vi "MetadataFromRD.vi"(9 "ChannelNames":string[](array[string]), 10 "ChannelName":string, 11 "Raw data file":path) -> (0 "allFound":bool, 1 "ValueStrings":string[](array[string]), 2 "ValueString":string, 4 "Name-Value Array":string[][](array[string]))   [LabVIEW 2021]
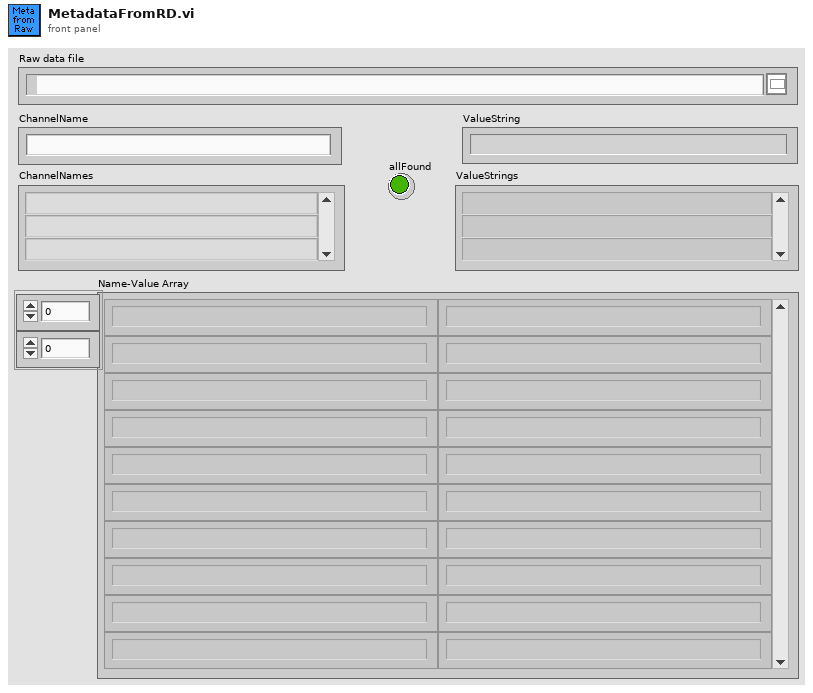
[diagram p1: front panel]
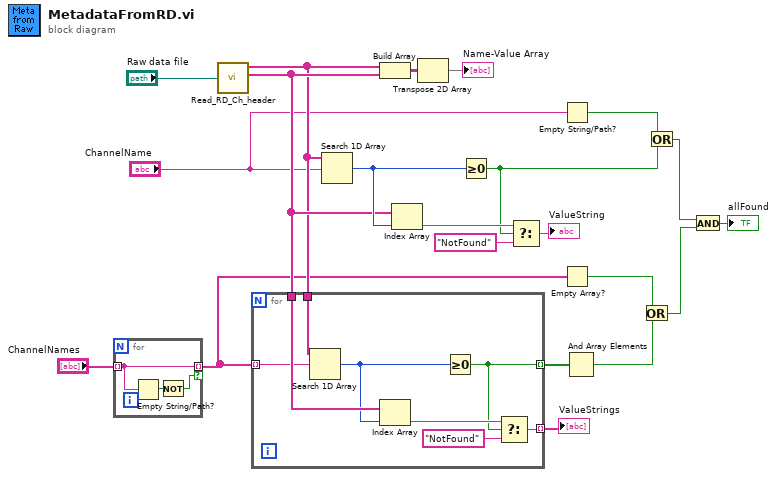
[diagram p0: block diagram]
diagram:
  n1 = for {
    tunnel: [w24] -> w2 mode=indexing if=w22
    tunnel: "ChannelNames" -> [w24] mode=indexing
    n2 = Empty String/Path?(string/path=w24) -> (empty?=w23:bool)
    n3 = Not(x=w23) -> (.not. x?=w22:bool)
  }
  n4 = call "Read_RD_Ch_header.vi"("Raw data file"="Raw data file") -> ("Ch Name Out"=w13:string[], "Ch Values"=w14:string[])  [unwired: 2 out]
  n5 = for {
    tunnel: w14 -> [w30]
    tunnel: w13 -> [w29]
    tunnel: w2 -> [w28] mode=indexing
    tunnel: [w27] -> w12 mode=indexing
    tunnel: [w25] -> w10 mode=indexing
    n6 = Search 1D Array(1D array=w29, element=w28) -> (index of element=w26:i32)  [unwired: 1 in]
    n7 = Index Array(array=w30, index=w26) -> (element=w32:string)
    n8 = Greater Or Equal To 0?(x=w26) -> (x >= 0?=w25:bool)
    n9 = Select(t=w32, s=w25, f="NotFound") -> (s? t:f=w27:string)
  }
  "ValueStrings" <- w12
  n10 = Search 1D Array(1D array=w13, element="ChannelName") -> (index of element=w18:i32)  [unwired: 1 in]
  n11 = Build Array(w13, w14) -> (w20:string[][])
  n12 = Index Array(array=w14, index=w18) -> (element=w16:string)
  n13 = Transpose 2D Array(2D array=w20) -> (transposed array=→"Name-Value Array":string[][])
  n14 = Greater Or Equal To 0?(x=w18) -> (x >= 0?=w8:bool)
  n15 = Select(t=w16, s=w8, f="NotFound") -> (s? t:f=→"ValueString":string)
  n16 = Empty String/Path?(string/path="ChannelName") -> (empty?=w9:bool)
  n17 = Empty Array?(array=w2) -> (empty?=w7:bool)
  n18 = And Array Elements(Boolean array=w10) -> (logical AND=w6:bool)
  n19 = Or(x=w7, y=w6) -> (x .or. y?=w4:bool)
  n20 = Or(x=w9, y=w8) -> (x .or. y?=w5:bool)
  n21 = And(x=w5, y=w4) -> (x .and. y?=→"allFound":bool)
